vi "TCP_Scratchpad.vi"(8 "error in (no error)":errorcluster, 11 "Cluster in":cluster{"Type":string, "Data":dbl[]}) -> (0 "error out":errorcluster, 3 "Cluster out":T1)   [LabVIEW 2026]
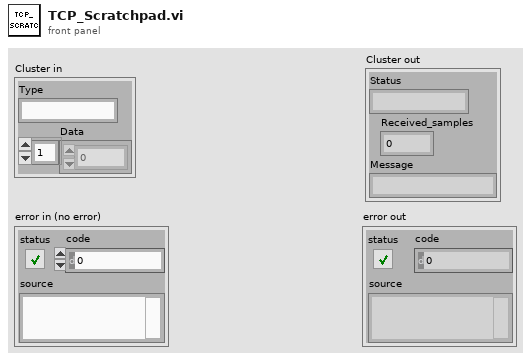
[diagram p1: front panel]
types:
  T1 = cluster{"Status":string, "Received_samples":i32, "Message":string}
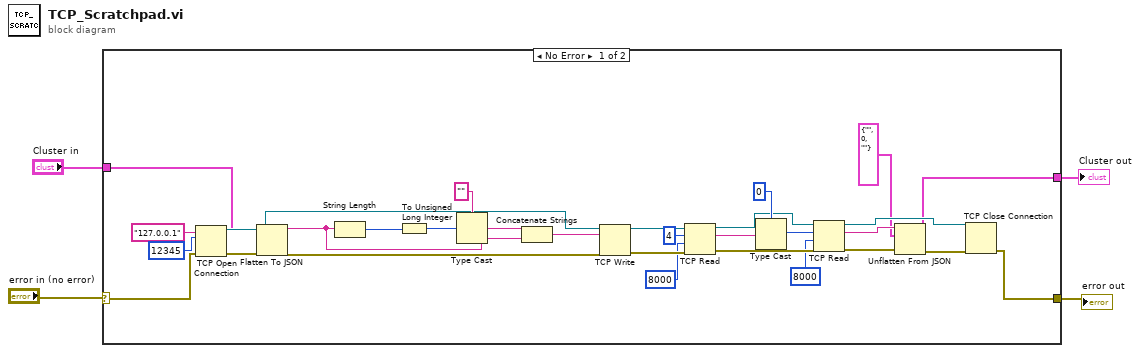
[diagram p0: block diagram]
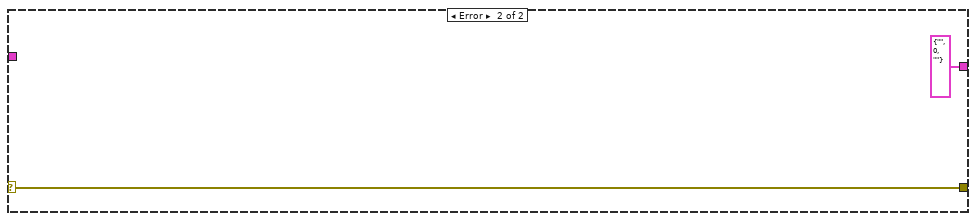
[diagram p2: hidden frame]
diagram:
  n1 = case shown="No Error" "error in (no error)" {
    selector: "error in (no error)" -> [w13 w36]
    tunnel: [w12 w36] -> w3
    tunnel: "Cluster in" -> [w6 _]
    tunnel: [w5 T1 {"Status"="", "Received_samples"=0, "Message"=""} ("Cluster 2")] -> w1
    frame No Error {
      n2 = TCP Open Connection(address="127.0.0.1", remote port or service name=u16 12345, error in (no error)=w13) -> (connection ID=w20:refnum<k5>, error out=w34:errorcluster)  [unwired: 2 in]
      n3 = Flatten To JSON(anything=w6, error in (no error)=w34) -> (JSON string=w31:string, 11:w29:errorcluster)  [unwired: 1 in]
      n4 = String Length(string=w31) -> (length=w9:i32)
      n5 = To Unsigned Long Integer(number=w9) -> (unsigned 32bit integer=w8:u32)
      n6 = Type Cast(type="", x=w8) -> (*(type *) &x=w32:string)
      n7 = Concatenate Strings(w32, w31) -> (w30:string)
      n8 = TCP Write(connection ID=w20, data in=w30, error in (no error)=w29) -> (connection ID out=w27:refnum<k5>, error out=w28:errorcluster)  [unwired: 1 in, 1 out]
      n9 = TCP Read(connection ID=w27, bytes to read=4, error in (no error)=w28, 9:8000 ("timeout ms (25000)")) -> (connection ID out=w19:refnum<k5>, data out=w26:string, error out=w17:errorcluster)  [unwired: 1 in]
      n10 = Type Cast(type=0 ("length"), x=w26) -> (*(type *) &x=w21:i32)
      n11 = TCP Read(connection ID=w19, bytes to read=w21, error in (no error)=w17, 9:8000 ("timeout ms (25000)")) -> (connection ID out=w18:refnum<k5>, data out=w24:string, error out=w23:errorcluster)  [unwired: 1 in]
      n12 = Unflatten From JSON(JSON string=w24, type and defaults=T1 {"Status"="", "Received_samples"=0, "Message"=""} ("Cluster 2"), error in (no error)=w23) -> (value=w5:T1, error out=w22:errorcluster)  [unwired: 4 in]
      n13 = TCP Close Connection(connection ID=w18, error in (no error)=w22) -> (error out=w12:errorcluster)  [unwired: 1 in, 1 out]
    }
    frame Error {
    }
  }
  "error out" <- w3
  "Cluster out" <- w1
